vi "Lock Control in The BottonCenter.vi"(6 "offset":cluster{"x":i32, "y":i32}, 8 "error in (no error)":errorcluster, 11 "TabControl in":refnum<vi>) -> (0 "error out":errorcluster)   [LabVIEW 2017]
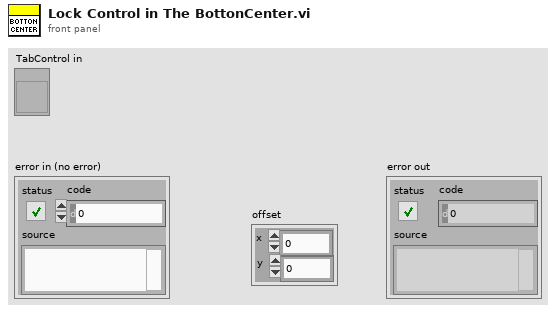
[diagram p1: front panel]
types:
  T1 = typedef "LVBoundsTypeDef.ctl" = cluster{"Width":u32, "Height":u32}
  T2 = typedef "LVPositionTypeDef.ctl" = cluster{"Left":i32, "Top":i32}
  T3 = cluster{"left":i16, "top":i16, "right":i16, "bottom":i16}
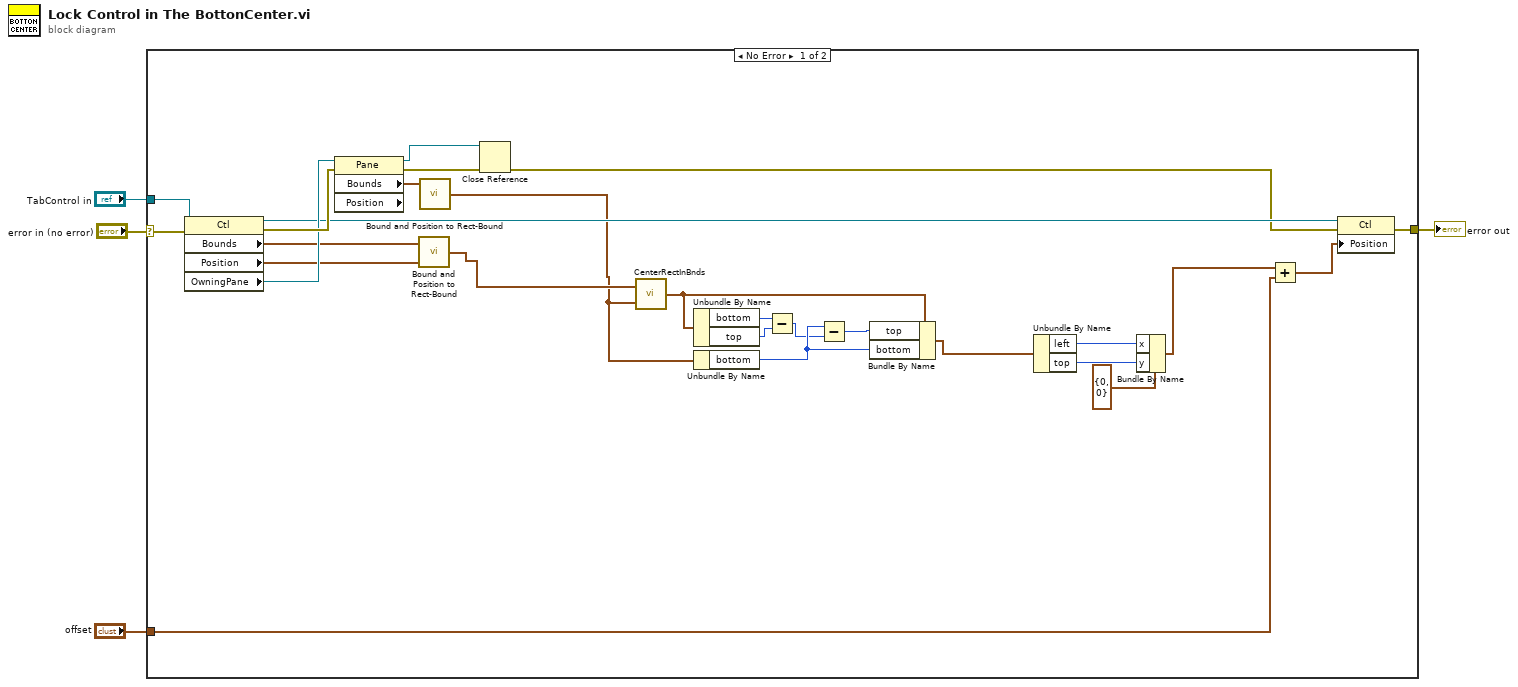
[diagram p0: block diagram]
diagram:
  n1 = case shown="No Error" "error in (no error)" {
    selector: "error in (no error)" -> [w20 w32]
    tunnel: "TabControl in" -> [w22 _]
    tunnel: [w21 w32] -> w3
    tunnel: "offset" -> [w19 _]
    frame No Error {
      n2 = property on="Property Node" class="Ctl"(reference=w22, error in=w20) -> (reference out=w28:refnum<vi>, error out=w30:errorcluster, "Bounds"=w23:T1, "Position"=w24:T2, "OwningPane"=w29:refnum<vi>)
      n3 = property on="Property Node" class="Pane" props=["Bounds", "Position"](reference=w29, error in=w30) -> (reference out=w14:refnum<vi>, error out=w31:errorcluster, "Bounds"=w25:T1)  [unwired: 1 out]
      n4 = call "Bound and Position to Rect-Bound.vi"("Position"=w24, "Bounds"=w23) -> ("Rect Bound"=w27:T3)  [unwired: 3 in]
      n5 = call "Bound and Position to Rect-Bound.vi"("Bounds"=w25) -> ("Rect Bound"=w26:T3)  [unwired: 4 in]
      n6 = Close Reference(reference=w14, error in (no error)=w31) -> (error out=w15:errorcluster)
      n7 = call <vilib>:"CenterRectInBnds.vi"("bounds"=w26, "rect"=w27) -> ("centered rect"=w13:T3)
      n8 = Unbundle By Name(w13) -> ("bottom"=w10:i16, "top"=w9:i16)
      n9 = Unbundle By Name(w26) -> ("bottom"=w11:i16)
      n10 = Subtract(x=w10, y=w9) -> (x-y=w8:i16)
      n11 = Subtract(x=w11, y=w8) -> (x-y=w12:i16)
      n12 = Bundle By Name(cluster=w13, "top"=w12, "bottom"=w11) -> (w18:T3)
      n13 = Unbundle By Name(w18) -> ("left"=w6:i16, "top"=w7:i16)
      n14 = Bundle By Name(cluster=cluster{"x":i32, "y":i32} {"x"=0, "y"=0} ("Point"), "x"=w6, "y"=w7) -> (w17:cluster{"x":i32, "y":i32})
      n15 = Add(x=w17, y=w19) -> (x+y=w16:cluster{"x":i32, "y":i32})
      n16 = property on="Property Node" class="Ctl"(reference=w28, error in=w15, "Position"=w16) -> (error out=w21:errorcluster)  [unwired: 1 out]
    }
    frame Error {
    }
  }
  "error out" <- w3
